vi "Write Numeric Value.vi"(8 "error in (no error)":errorcluster, 10 "Numeric Value":dbl, 11 "Numeric Assertion in":refnum<class "Numeric Assertion.lvclass">) -> (0 "error out":errorcluster, 3 "Numeric Assertion out":refnum<class "Numeric Assertion.lvclass">)   [LabVIEW 2020, in "MacroAssert.lvlib" / "Numeric Assertion.lvclass"]
uses:
  Numeric Assertion.lvclass
  Numeric Assertion.lvclass/Numeric Assertion.ctl
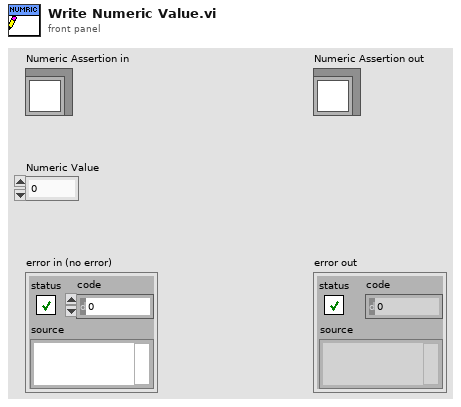
[diagram p1: front panel]
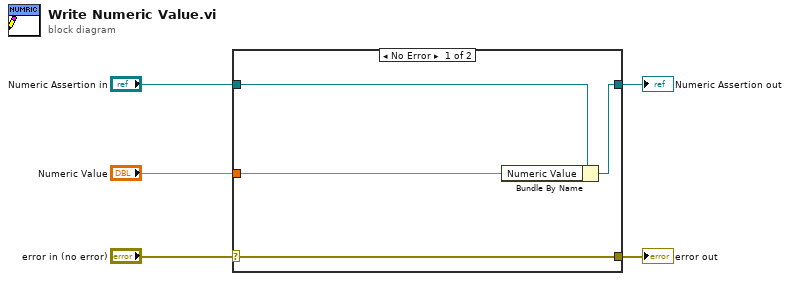
[diagram p0: block diagram]
diagram:
  n1 = case shown="No Error" "error in (no error)" {
    selector: "error in (no error)" -> [w9 w10]
    tunnel: [w9 w10] -> w4
    tunnel: [w7 w11] -> w2
    tunnel: "Numeric Assertion in" -> [w8 w11]
    tunnel: "Numeric Value" -> [w6 _]
    frame No Error {
      n2 = Bundle By Name(cluster=w8, "Numeric Value"=w6) -> (w7:refnum<class "Numeric Assertion.lvclass">)
    }
    frame Error {
    }
  }
  "error out" <- w4
  "Numeric Assertion out" <- w2
